vi "DC_Overvoltage_v1.vi"(8 "error in":errorcluster) -> (0 "error out":errorcluster, 3 "Result":dbl[](array[numeric]))   [LabVIEW 2022 SP3]
uses:
  <vilib>/DAQmx/write.llb/DAQmx Write (Analog 1D DBL NChan 1Samp).vi
  <vilib>/DAQmx/read.llb/DAQmx Read (Analog DBL 1Chan 1Samp).vi
  <vilib>/DAQmx/miscellaneous.llb/DAQmx Fill In Error Info.vi
panel:
  in  "Starting Voltage":dbl
  in  "Latch Low Threshold":dbl
  out "VDC Unlatch":dbl[](array[numeric])
  out "V_Fault Unlatch":dbl format="%0.2f"
  out "V_Fault Latch":dbl format="%0.2f"
  in  "Max Voltage":dbl
  out "VDC Latch":dbl[](array[numeric])
  in  "Increments":i32
  in  "Latch High Threshold":dbl
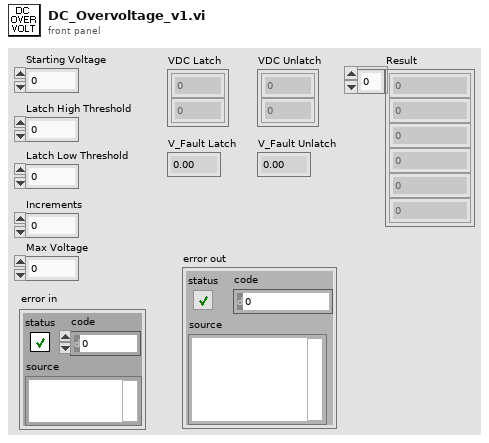
[diagram p1: front panel]
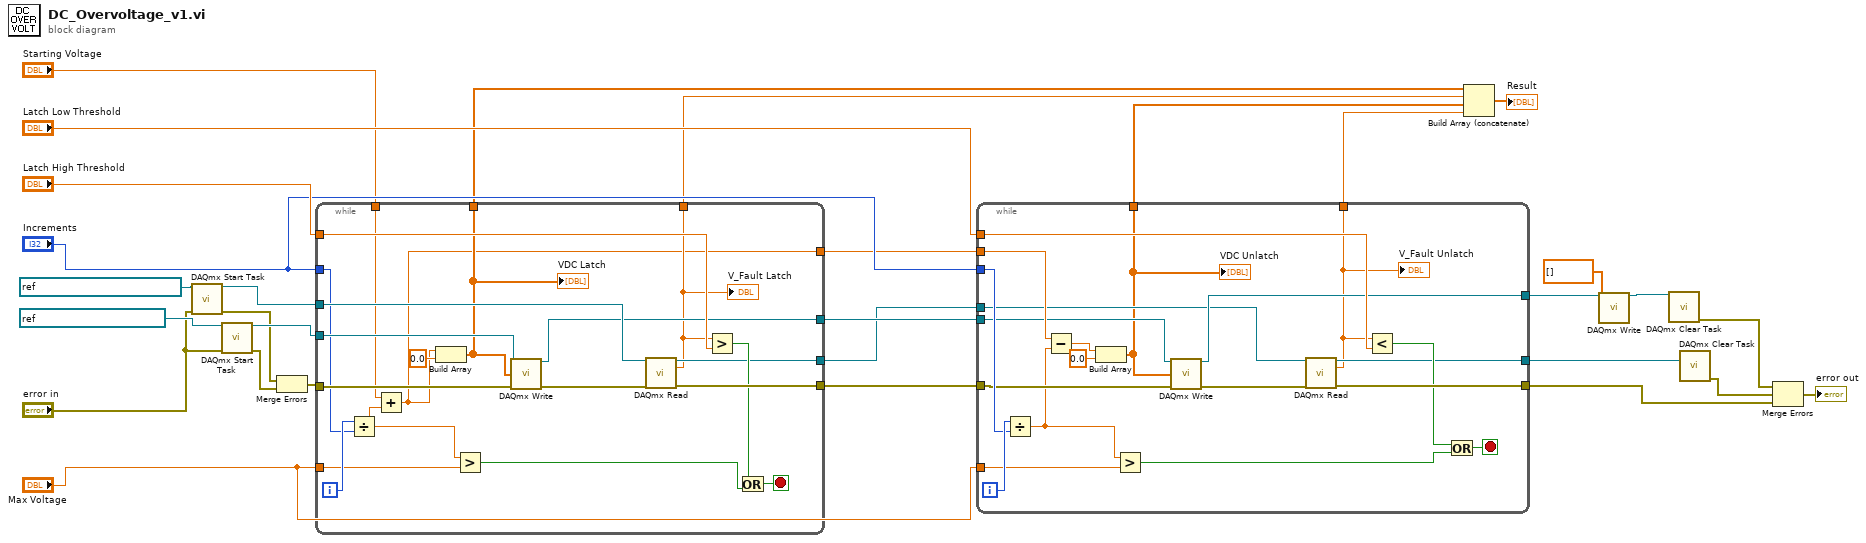
[diagram p0: block diagram]
diagram:
  n1 = call <vilib>:"DAQmx Start Task.vi"("task/channels in"=refnum<k21> "BONTS-DC-OV-Feedback", "error in"="error in") -> ("task out"=w27:refnum<k21>, "error out"=w17:errorcluster)  [unwired: 12 in]
  n2 = call <vilib>:"DAQmx Start Task.vi"("task/channels in"=refnum<k21> "BONTS_DC-Link_Input", "error in"="error in") -> ("task out"=w29:refnum<k21>, "error out"=w16:errorcluster)  [unwired: 12 in]
  n3 = Merge Errors(w17, w16) -> (w18:errorcluster)
  n4 = while {
    tunnel: w27 -> [w50]
    tunnel: w29 -> [w49]
    tunnel: w18 -> [w48]
    tunnel: [w47] -> w13
    tunnel: "Latch High Threshold" -> [w45]
    tunnel: "Increments" -> [w43]
    tunnel: "Max Voltage" -> [w41]
    tunnel: [w37] -> w12
    tunnel: [w36] -> w11
    tunnel: [w32] -> w10
    tunnel: [w35] -> w6
    tunnel: [w34] -> w7
    tunnel: "Starting Voltage" -> [w31]
    i -> [w44]
    stop <- w38 stop-if-true
    n5 = Divide(x=w44, y=w43) -> (x/y=w33:dbl)
    n6 = Add(x=w31, y=w33) -> (x+y=w32:dbl)
    n7 = Build Array(w32, 0.0 ("element")) -> (w35:dbl[])
    "VDC Latch" <- w35
    n8 = Greater?(x=w33, y=w41) -> (0:w39:bool)
    n9 = call-poly <vilib>:"DAQmx Write.vi"("task/channels in"=w49, "data"=w35, "error in"=w48) -> ("task out"=w37:refnum<k21>, "error out"=w46:errorcluster)  [unwired: 10 in, 1 out]
    n10 = call-poly <vilib>:"DAQmx Read.vi"("task/channels in"=w50, "error in"=w46) -> ("task out"=w36:refnum<k21>, "data"=w34:dbl, "error out"=w47:errorcluster)  [unwired: 11 in]
    "V_Fault Latch" <- w34
    n11 = Greater?(x=w34, y=w45) -> (0:w40:bool)
    n12 = Or(x=w40, y=w39) -> (x .or. y?=w38:bool)
  }
  n13 = while {
    tunnel: [w70] -> w20
    tunnel: "Latch Low Threshold" -> [w68]
    tunnel: "Increments" -> [w66]
    tunnel: "Max Voltage" -> [w64]
    tunnel: [w60] -> w23
    tunnel: [w59] -> w3
    tunnel: w13 -> [w58]
    tunnel: w10 -> [w55]
    tunnel: w12 -> [w54]
    tunnel: w11 -> [w53]
    tunnel: [w52] -> w8
    tunnel: [w51] -> w9
    i -> [w67]
    stop <- w61 stop-if-true
    n14 = Divide(x=w67, y=w66) -> (x/y=w56:dbl)
    n15 = Subtract(x=w55, y=w56) -> (x-y=w57:dbl)
    n16 = Build Array(w57, 0.0 ("element")) -> (w52:dbl[])
    "VDC Unlatch" <- w52
    n17 = Greater?(x=w56, y=w64) -> (0:w62:bool)
    n18 = call-poly <vilib>:"DAQmx Write.vi"("task/channels in"=w54, "data"=w52, "error in"=w58) -> ("task out"=w59:refnum<k21>, "error out"=w69:errorcluster)  [unwired: 10 in, 1 out]
    n19 = call-poly <vilib>:"DAQmx Read.vi"("task/channels in"=w53, "error in"=w69) -> ("task out"=w60:refnum<k21>, "data"=w51:dbl, "error out"=w70:errorcluster)  [unwired: 11 in]
    "V_Fault Unlatch" <- w51
    n20 = Less?(x=w51, y=w68) -> (x < y?=w63:bool)
    n21 = Or(x=w63, y=w62) -> (x .or. y?=w61:bool)
  }
  n22 = Build Array (concatenate)(w6, w7, w8, w9) -> (→"Result":dbl[])
  n23 = call-poly <vilib>:"DAQmx Write.vi"("task/channels in"=w3, "data"=dbl[] []) -> ("task out"=w2:refnum<k21>)  [unwired: 11 in, 2 out]
  n24 = call <vilib>:"DAQmx Clear Task.vi"("task in"=w2) -> ("error out"=w22:errorcluster)  [unwired: 14 in]
  n25 = call <vilib>:"DAQmx Clear Task.vi"("task in"=w23) -> ("error out"=w21:errorcluster)  [unwired: 14 in]
  n26 = Merge Errors(w22, w21, w20) -> (→"error out":errorcluster)
